vi "VeriStand FPGA Wizard.vi"() -> ()   [LabVIEW 2015]
uses:
  Classes/Project/Project.lvclass
panel:
  in  "WebBrowser":refnum<k7>(container)
  in  "Export":bool
  in  "error in":errorcluster
  in  "Exit":bool
  in  "Build":bool
  in  "IO CSV Path":path
  in  "Project Path":path
  out "error out":errorcluster
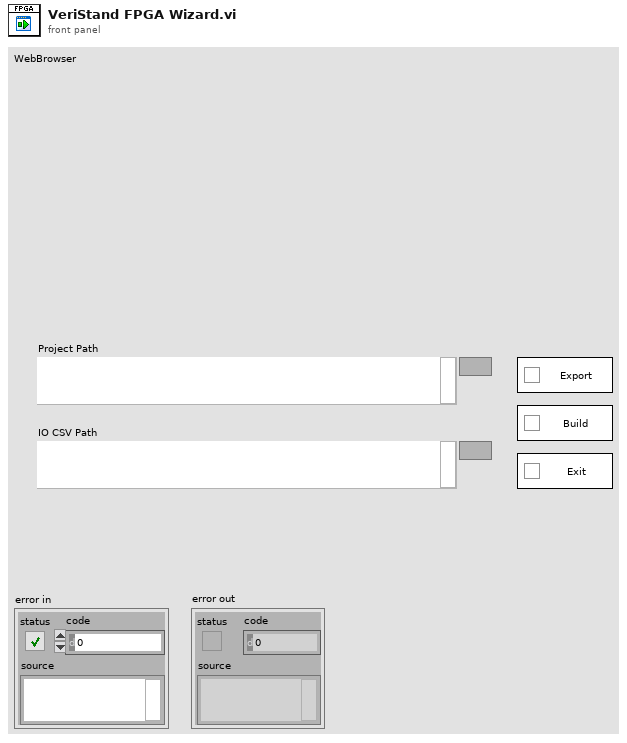
[diagram p1: front panel]
types:
  T1 = typedef "Project.lvclass/FPGA Settings.ctl" = cluster{"FPGA Target Name":string, "Modules":T2[]}
  T2 = typedef "Module.lvclass/Module Settings.ctl" = cluster{"Group Name":string, "Model Number":string, "Signals":T3[]}
  T3 = typedef "Signal.lvclass/Signal Settings.ctl" = cluster{"Signal Name":string, "IO Name":string, "Signal Type":string, "Signal Parameters":string, "IO Resource":string}
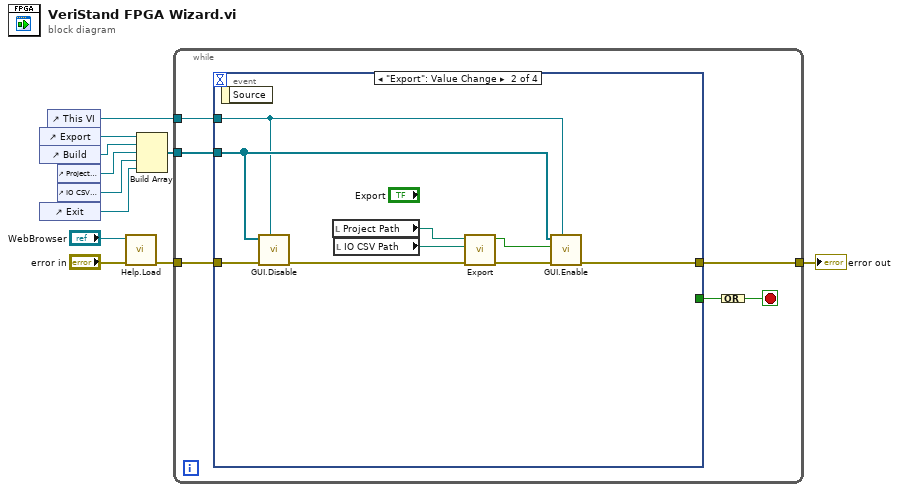
[diagram p0: block diagram]
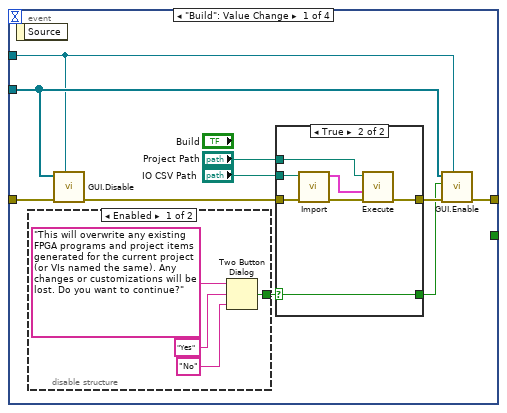
[diagram p2: hidden frame]
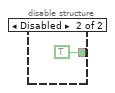
[diagram p3: hidden frame]
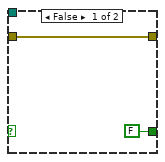
[diagram p4: hidden frame]
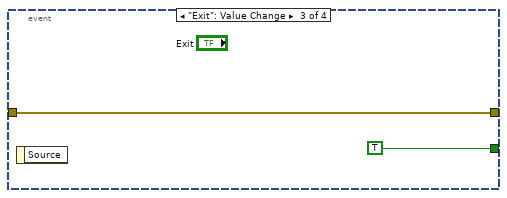
[diagram p5: hidden frame]
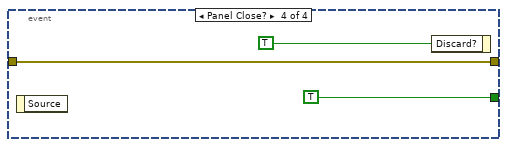
[diagram p6: hidden frame]
diagram:
  n1 = control-ref of="Export"() -> (w1:refnum<vi>)
  n2 = control-ref of="Build"() -> (w10:refnum<vi>)
  n3 = control-ref of="Exit"() -> (w7:refnum<vi>)
  n4 = control-ref of="This VI"() -> (w2:refnum<vi>)
  n5 = control-ref of="Project Path"() -> (w9:refnum<vi>)
  n6 = control-ref of="IO CSV Path"() -> (w8:refnum<vi>)
  n7 = call "Help.Load.vi"("error in (no error)"="error in", "Web Browser Reference"="WebBrowser") -> ("error out"=w4:errorcluster)  [unwired: 9 in]
  n8 = Build Array(w1, w10, w9, w8, w7) -> (w6:refnum<vi>[])
  n9 = while {
    tunnel: w6 -> [w14]
    tunnel: w2 -> [w13]
    tunnel: w4 -> [w17]
    tunnel: [w12] -> w11
    stop <- w15 stop-if-true
    n10 = event shown="[1] \"Export\": Value Change" {
      selector: _ -> [_ _ _ _]
      dyn-events: _ -> [_ _ _ _]
      timeout: _ -> [_ _ _ _]
      tunnel: [w21 w48 w52 w55] -> w12
      tunnel: w17 -> [w22 w49 w52 w55]
      tunnel: [_ _ TRUE TRUE] -> w16
      tunnel: w14 -> [w23 w50 _ _]
      tunnel: w13 -> [w20 w43 _ _]
      event "Build": Value Change {
        n11 = event-data() -> ()  [unwired: 1 in, 1 out]
        n12 = disable-structure shown="Enabled" {
          disable-tunnel: [w28 TRUE ("T button?")] -> w19
          frame Enabled {
            n13 = Two Button Dialog(message="This will overwrite any existing FPGA programs and project items generated for the current project (or VIs named the same). Any changes or customizations will be lost. Do you want to continue?", 1:"No" ("F button name (\"Cancel\")"), 2:"Yes" ("T button name (\"OK\")")) -> (T button?=w28:bool)
          }
          frame Disabled {
          }
        }
        n14 = call "GUI.Disable.vi"("VI reference (current VI)"=w20, "error in (no error)"=w22, "Array"=w23) -> ("error out"=w25:errorcluster)  [unwired: 8 in]
        n15 = case shown="True" w19 {
          selector: w19 -> [_ w35]
          tunnel: "Project Path" -> [_ w41]
          tunnel: "IO CSV Path" -> [_ w38]
          tunnel: w25 -> [w34 w37]
          tunnel: [w34 w36] -> w24
          tunnel: [FALSE w35] -> w18
          frame False {
          }
          frame True {
            n16 = call "Import.vi"("error in"=w37, "CSV Path"=w38) -> ("error out"=w40:errorcluster, "FPGA Settings"=w39:T1[])  [unwired: 8 in]
            n17 = call "Execute.vi"("error in (no error)"=w40, "Targets"=w39, "Project Path"=w41) -> ("error out"=w36:errorcluster)  [unwired: 8 in]
          }
        }
        n18 = call "GUI.Enable.vi"("VI reference (current VI)"=w20, "error in (no error)"=w24, "Ran?"=w18, "Array"=w23) -> ("error out"=w21:errorcluster)  [unwired: 7 in]
      }
      event "Export": Value Change {
        n19 = event-data() -> ()  [unwired: 1 in, 1 out]
        n20 = call "GUI.Disable.vi"("VI reference (current VI)"=w43, "error in (no error)"=w49, "Array"=w50) -> ("error out"=w45:errorcluster)  [unwired: 8 in]
        n21 = local read "Project Path"() -> (w47:path)
        n22 = local read "IO CSV Path"() -> (w46:path)
        n23 = call "Export.vi"("error in (no error)"=w45, "Export Path"=w46, "Project Path"=w47) -> ("error out"=w44:errorcluster, "Ran?"=w42:bool)  [unwired: 7 in]
        n24 = call "GUI.Enable.vi"("VI reference (current VI)"=w43, "error in (no error)"=w44, "Ran?"=w42, "Array"=w50) -> ("error out"=w48:errorcluster)  [unwired: 7 in]
      }
      event "Exit": Value Change {
        n25 = event-data() -> ()  [unwired: 1 in, 1 out]
      }
      event Panel Close? {
        n26 = event-data() -> ()  [unwired: 1 in, 1 out]
        n27 = event-data("Discard?"=TRUE) -> ()  [unwired: 1 in, 1 out]
      }
    }
    n28 = Compound Arithmetic op=OR(w16) -> (w15:bool)
  }
  "error out" <- w11
